vi "SerialPort.Set Status Control State.vi"(8 "error in (no error)":errorcluster, 11 "SerialPort in":refnum<class "SerialPort.lvclass">) -> (0 "error out":errorcluster, 3 "SerialPort out":refnum<class "SerialPort.lvclass">)   [LabVIEW 2018, in "SerialPort.lvclass"]
uses:
  SerialPort.lvclass
  SerialPort.lvclass/SerialPort.ctl
panel:
  out "Updated":bool
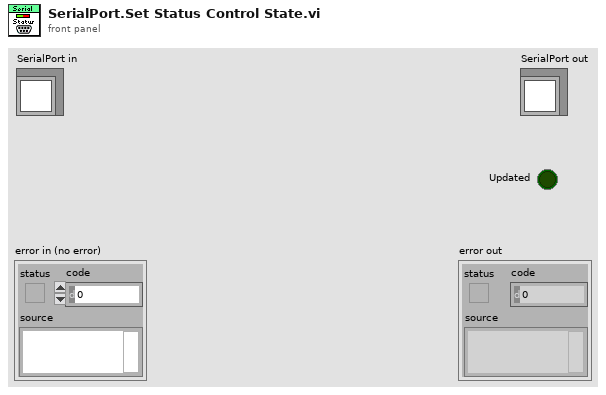
[diagram p1: front panel]
types:
  T1 = typedef "SerialPort.Status Enum.ctl" = enum16{"Disconnected", "Connecting", "Connected"}
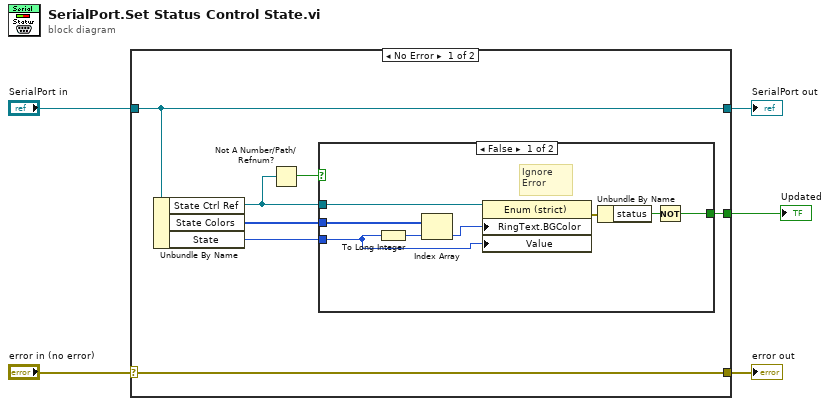
[diagram p0: block diagram]
diagram:
  n1 = case shown="No Error" "error in (no error)" {
    selector: "error in (no error)" -> [w12 w22]
    tunnel: [w12 w22] -> w4
    tunnel: [w9 w21] -> w2
    tunnel: "SerialPort in" -> [w9 w21]
    tunnel: [w6 _] -> w1
    frame No Error {
      n2 = Unbundle By Name(w9) -> ("State Ctrl Ref"=w8:refnum<vi>, "State Colors"=w11:u32[], "State"=w10:T1)
      n3 = Not A Number/Path/Refnum?(number/path/refnum=w8) -> (NaN/Path/Refnum?=w7:bool)
      n4 = case shown="False" w7 {
        tunnel: w11 -> [w19 _]
        tunnel: w10 -> [w17 _]
        tunnel: w8 -> [w16 _]
        tunnel: [w13 _] -> w6
        frame False {
          # "Ignore\nError"
          n5 = To Long Integer(number=w17) -> (32bit integer=w20:i32)
          n6 = Index Array(array=w19, index=w20) -> (element=w18:u32)
          n7 = property class="Enum (strict)"(reference=w16, "RingText.BGColor"=w18, "Value"=w17) -> (error out=w15:errorcluster)  [unwired: 1 in, 1 out]
          n8 = Unbundle By Name(w15) -> ("status"=w14:bool)
          n9 = Not(x=w14) -> (.not. x?=w13:bool)
        }
        frame True {
          # "Control ref is not configured\nDo nothing"
        }
      }
    }
    frame Error {
    }
  }
  "error out" <- w4
  "SerialPort out" <- w2
  "Updated" <- w1
